vi "Open Preference File.vi"(4 "error In":errorcluster, 6 "Initialize":bool, 7 "Server":bool) -> (0 "error":errorcluster, 2 "ipf path":path, 3 "refnum":T1)   [LabVIEW 2018]
uses:
  <vilib>/Utility/config.llb/Config Data RefNum.ctl
  <vilib>/Utility/config.llb/NI_LVConfig.lvlib
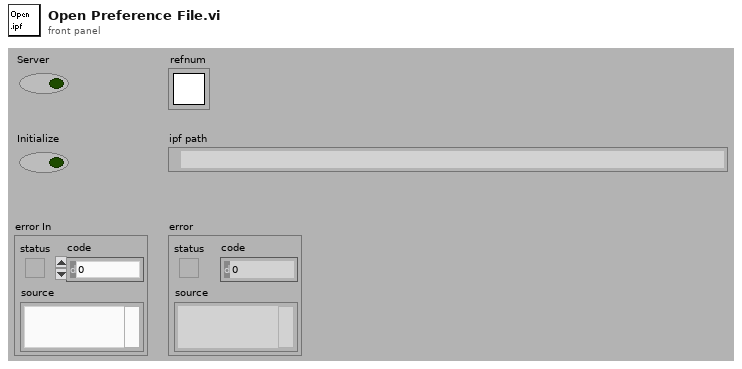
[diagram p1: front panel]
types:
  T1 = typedef "NI_LVConfig.lvlib/Config Data RefNum.ctl" = refnum<k1>
  T2 = enum32{"existing file", "new file", "new or existing file", "existing dir", "new dir", "new or existing dir", "existing file (use LLBs)", "new file (use LLBs)", "new or existing file (use LLBs)", "new or existing file or directory (use LLBs)"}
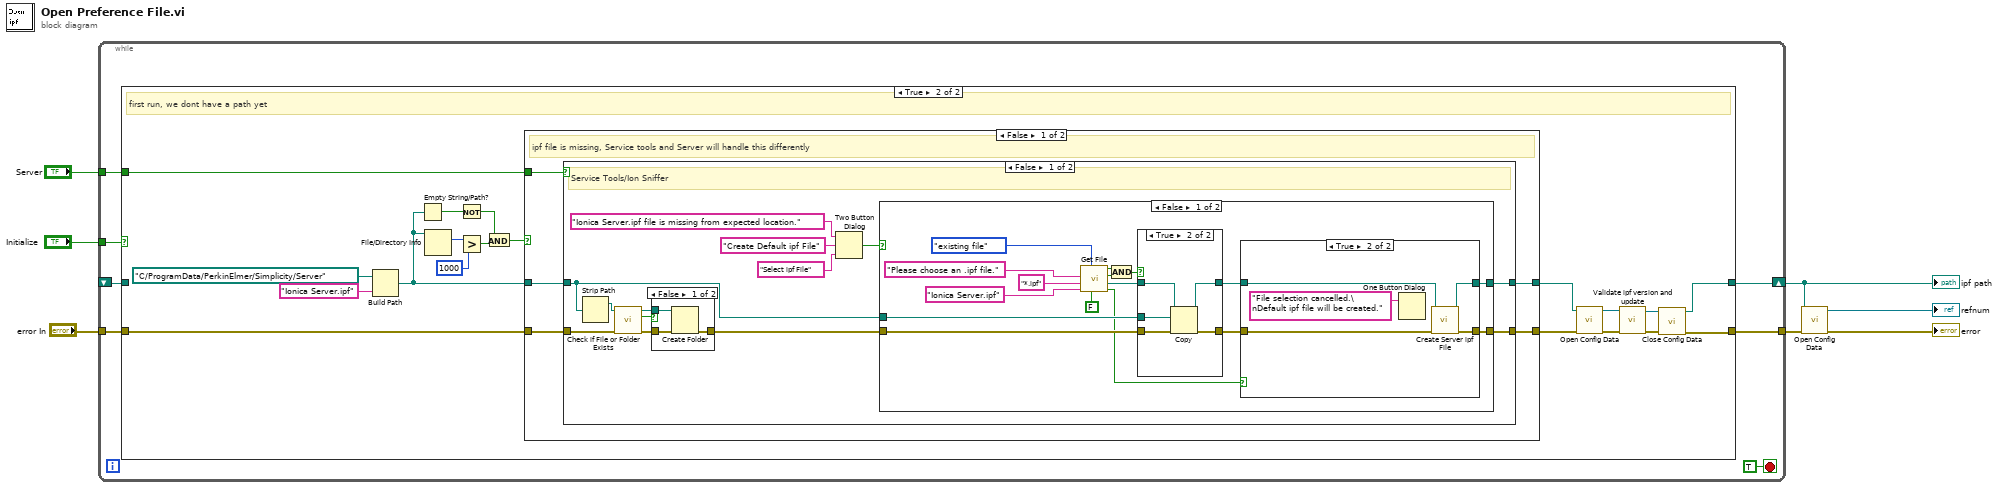
[diagram p0: block diagram]
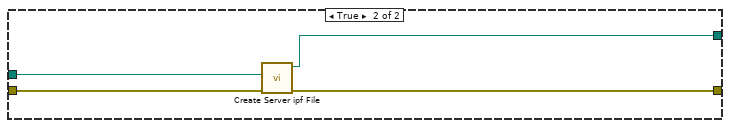
[diagram p5: hidden frame]
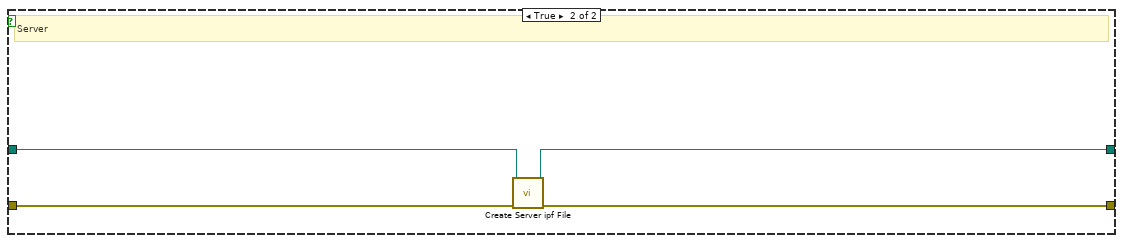
[diagram p7: hidden frame]
diagram:
  n1 = while {
    tunnel: "Server" -> [w13]
    shift-right: [w14] -> w7
    shift-left: _ -> [w10]
    tunnel: "Initialize" -> [w12]
    tunnel: "error In" -> [w9]
    tunnel: [w8] -> w3
    stop <- TRUE stop-if-true
    n2 = case shown="True" w12 {
      tunnel: [w16 w22] -> w14
      tunnel: w13 -> [_ w25]
      tunnel: w10 -> [w16 _]
      tunnel: w9 -> [w15 w26]
      tunnel: [w15 w23] -> w8
      frame False {
        # "we already have a file path, use it"
      }
      frame True {
        # "first run, we dont have a path yet"
        n3 = Build Path(base path=path "C:/ProgramData/PerkinElmer/Simplicity/Server" ("appended path"), name or relative path="Ionica Server.ipf") -> (appended path=w33:path)
        n4 = Empty String/Path?(string/path=w33) -> (empty?=w29:bool)
        n5 = File/Directory Info(path=w33) -> (size=w31:i64)  [unwired: 1 in, 6 out]
        n6 = Not(x=w29) -> (.not. x?=w30:bool)
        n7 = Greater?(x=w31, y=i64 1000) -> (0:w28:bool)
        n8 = And(x=w30, y=w28) -> (x .and. y?=w27:bool)
        n9 = case shown="False" w27 {
          tunnel: [w40 w97] -> w21
          tunnel: w33 -> [w39 w97]
          tunnel: w25 -> [w38 _]
          tunnel: w26 -> [w37 w96]
          tunnel: [w36 w96] -> w24
          frame False {
            # "ipf file is missing, Service tools and Server will handle this differently"
            n10 = case shown="False" w38 {
              tunnel: [w45 w94] -> w40
              tunnel: w39 -> [w48 w95]
              tunnel: w37 -> [w53 w93]
              tunnel: [w46 w92] -> w36
              frame False {
                # "Service Tools/Ion Sniffer"
                n11 = Strip Path(path=w48) -> (stripped path=w47:path)  [unwired: 1 out]
                n12 = call <vilib>:"Check if File or Folder Exists.vi"("error in (no error)"=w53, "path"=w47) -> ("error out"=w52:errorcluster, "file or folder exists?"=w49:bool, "dup path"=w50:path)  [unwired: 7 in]
                n13 = case shown="False" w49 {
                  tunnel: w52 -> [w90 w91]
                  tunnel: [w89 w91] -> w51
                  tunnel: w50 -> [w88 _]
                  frame False {
                    n14 = Create Folder(path (use dialog)=w88, error in=w90) -> (error out=w89:errorcluster)  [unwired: 1 in, 2 out]
                  }
                  frame True {
                  }
                }
                n15 = Two Button Dialog(message="Ionica Server.ipf file is missing from expected location.", 1:"Select ipf File" ("T button name (\"OK\")"), 2:"Create Default ipf File" ("T button name (\"OK\")")) -> (T button?=w41:bool)
                n16 = case shown="False" w41 {
                  tunnel: w51 -> [w60 w87]
                  tunnel: w48 -> [w59 w85]
                  tunnel: [w57 w86] -> w46
                  tunnel: [w55 w84] -> w45
                  frame False {
                    n17 = call "Get File.vi"("For Write (T)"=FALSE, "select mode (new or existing)"=T2."existing file", "default name"="Ionica Server.ipf", "extension (isd)"="*.ipf", "prompt"="Please choose an .ipf file.") -> ("cancelled"=w54:bool, "Seleted File"=w61:path, "Exists"=w63:bool, "Succeeded"=w64:bool)  [unwired: 1 in]
                    n18 = And(x=w64, y=w63) -> (x .and. y?=w62:bool)
                    n19 = case shown="True" w62 {
                      tunnel: w61 -> [_ w83]
                      tunnel: w59 -> [w78 w82]
                      tunnel: [w78 w81] -> w56
                      tunnel: w60 -> [w77 w80]
                      tunnel: [w77 w79] -> w58
                      frame False {
                      }
                      frame True {
                        n20 = Copy(8:w80, 10:w82, 11:w83) -> (0:w79:errorcluster, 3:w81:path)  [unwired: 2 in, 1 out]
                      }
                    }
                    n21 = case shown="True" w54 {
                      tunnel: w58 -> [w71 w76]
                      tunnel: [w71 w75] -> w57
                      tunnel: w56 -> [w70 w74]
                      tunnel: [w70 w73] -> w55
                      frame False {
                      }
                      frame True {
                        n22 = One Button Dialog(message="File selection cancelled.\nDefault ipf file will be created.") -> ()  [unwired: 1 in, 1 out]
                        n23 = call "Create Server ipf File.vi"("error in"=w76, "Default ipf file path"=w74) -> ("error out"=w75:errorcluster, "ipf file path"=w73:path)  [unwired: 8 in]
                      }
                    }
                  }
                  frame True {
                    n24 = call "Create Server ipf File.vi"("error in"=w87, "Default ipf file path"=w85) -> ("error out"=w86:errorcluster, "ipf file path"=w84:path)  [unwired: 8 in]
                  }
                }
              }
              frame True {
                # "Server"
                n25 = call "Create Server ipf File.vi"("error in"=w93, "Default ipf file path"=w95) -> ("error out"=w92:errorcluster, "ipf file path"=w94:path)  [unwired: 8 in]
              }
            }
          }
          frame True {
            # ".ipf File found use it"
          }
        }
        n26 = call <vilib>:"Open Config Data.vi"("error in (no error)"=w24, "configuration file path"=w21) -> ("error out"=w19:errorcluster, "refnum"=w20:T1)  [unwired: 7 in, 1 out]
        n27 = call "Validate ipf version and update.vi"("error In"=w19, "refnum In"=w20) -> ("error Out"=w18:errorcluster, "refnum Out"=w17:T1)  [unwired: 8 in]
        n28 = call <vilib>:"Close Config Data.vi"("error in (no error)"=w18, "refnum"=w17) -> ("error out"=w23:errorcluster, "file path"=w22:path)  [unwired: 8 in]
      }
    }
  }
  "ipf path" <- w7
  n29 = call <vilib>:"Open Config Data.vi"("error in (no error)"=w3, "configuration file path"=w7) -> ("error out"=→"error":errorcluster, "refnum"=→"refnum":T1)  [unwired: 7 in, 1 out]
